vi "checkFreqTemp.vi"(1 "Path":path, 4 "Temp":dbl, 5 "Error Temp":dbl, 6 "error in":errorcluster, 7 "Set Frequency":dbl) -> (0 "error out":errorcluster, 2 "Amplitude":dbl, 3 "Phase Shift":dbl)   [LabVIEW 2010]
uses:
  <vilib>/Utility/file.llb/Write To Spreadsheet File (DBL).vi
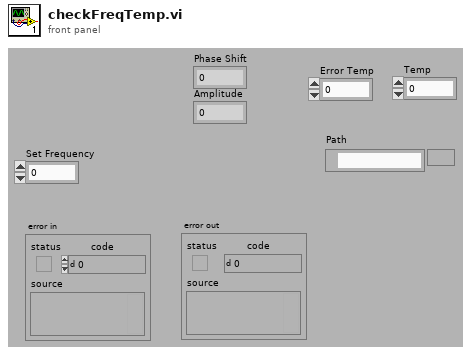
[diagram p1: front panel]
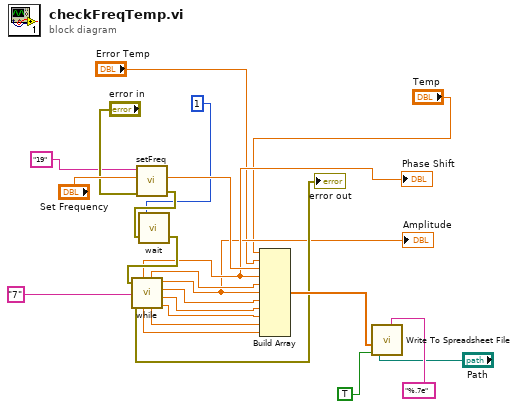
[diagram p0: block diagram]
diagram:
  n1 = call "setFreq.vi"("error in"="error in", "Frequenz in Hz"="Set Frequency", "address string"="19") -> ("error out"=w15:errorcluster)  [unwired: 3 in]
  n2 = call "wait.vi"("error in"=w15, "Wartezeit in Sek"=1) -> ("error out"=w14:errorcluster)  [unwired: 1 in]
  n3 = call "while.vi"("error in"=w14, "adress string"="7") -> ("Phase Shift"=w6:dbl, "error out"=→"error out":errorcluster, "Errror U2"=w12:dbl, "Error PS"=w7:dbl, "Amplitude"=w5:dbl, "Error  Amp"=w8:dbl, "U2"=w11:dbl, "U1"=w9:dbl, "Error U1"=w10:dbl)
  "Phase Shift" <- w6
  "Amplitude" <- w5
  n4 = Build Array("Temp", "Error Temp", "Set Frequency", w6, w7, w5, w8, w9, w10, w11, w12) -> (w20:dbl[])
  n5 = call-poly <vilib>:"Write To Spreadsheet File.vi"("format (%.3f)"="%.7e", "append to file? (new file:F)"=TRUE, "1D data"=w20, "file path (dialog if empty)"="Path") -> ()  [unwired: 4 in, 1 out]
